vi "SP Find Limit by Parameter.vi"(10 "Parameter":T1={"Stimulus Port"=1, "Response Port"=1} caption="Parameter String" {"Stimulus Port" min=1 step=1; "Response Port" min=1 step=1}, 11 "Limits":T2[](array[typedef]) {"Parameter"."Stimulus Port" min=1 step=1; "Parameter"."Response Port" min=1 step=1}) -> (0 "Found?":bool, 3 "Limits":T2[](array[typedef]) {"Parameter"."Stimulus Port" min=1 step=1; "Parameter"."Response Port" min=1 step=1})   [LabVIEW 2011]
uses:
  TypeDefs/SP Limit.ctl
  TypeDefs/SP Parameter.ctl
  TypeDefs/SP Format.ctl
  TypeDefs/SP Limit Type.ctl
  TypeDefs/SP Limit Point.ctl
  Test Referential Limit.ctl
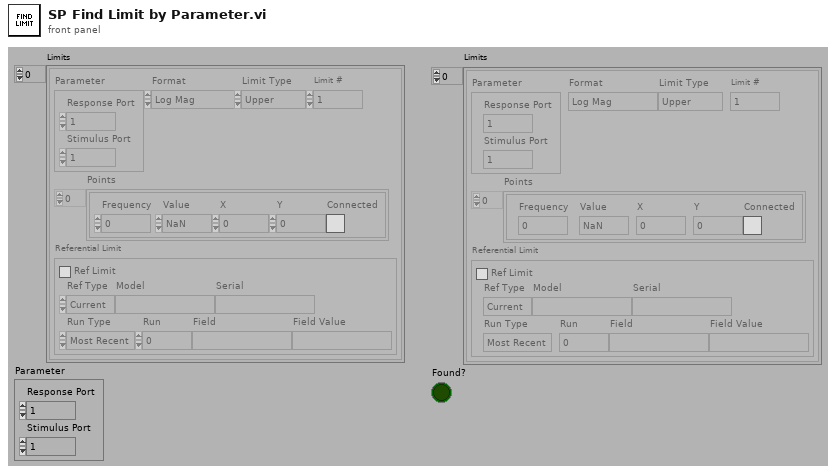
[diagram p1: front panel]
types:
  T1 = typedef "SP Parameter.ctl" = cluster{"Stimulus Port":i8, "Response Port":i8}
  T2 = typedef "SP Limit.ctl" = cluster{"Parameter":T1, "Format":T3, "Limit Type":T4, "Points":T5[], "Referential Limit":T6, "Limit #":i8}
  T3 = typedef "SP Format.ctl" = enum16{"Log Mag", "Lin Mag", "SWR", "Phase", "Expanded Phase", "Delay", "Insertion Loss", "Isolation", "Return Loss"}
  T4 = typedef "SP Limit Type.ctl" = enum16{"Upper", "Lower", "Delta", "Filter", "Referential"}
  T5 = typedef "SP Limit Point.ctl" = cluster{"Frequency":dbl, "Value":dbl, "X":dbl, "Y":dbl, "Connected":bool}
  T6 = typedef "Test Referential Limit.ctl" = cluster{"Ref Limit":bool, "Ref Type":enum16{"Current", "Specify"}, "Model":string, "Serial":string, "Run Type":enum16{"Most Recent", "Run #", "Match Field"}, "Run":i32, "Field":string, "Field Value":string}
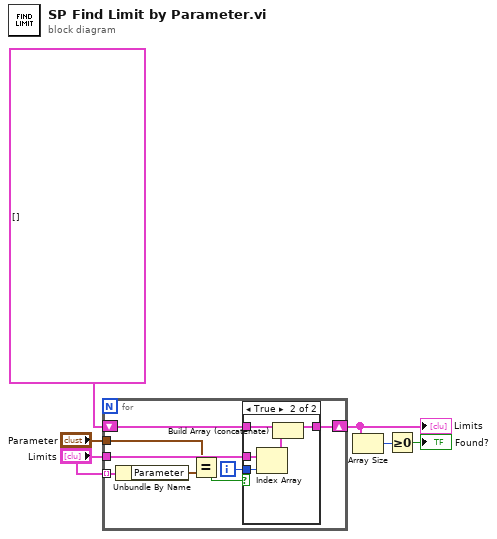
[diagram p0: block diagram]
diagram:
  n1 = for {
    tunnel: "Limits" -> [w14] mode=indexing
    tunnel: "Limits" -> [w13]
    shift-right: [w10] -> w4
    shift-left: T2[] [] ("Limits") -> [w11]
    tunnel: "Parameter" -> [w8]
    i -> [w12]
    n2 = Unbundle By Name(w14) -> ("Parameter"=w9:T1)
    n3 = Equal?(x=w8, y=w9) -> (x = y?=w7:bool)
    n4 = case shown="True" w7 {
      tunnel: w13 -> [_ w20]
      tunnel: w12 -> [_ w19]
      tunnel: w11 -> [w15 w17]
      tunnel: [w15 w16] -> w10
      frame False {
      }
      frame True {
        n5 = Index Array(array=w20, index=w19) -> (element=w18:T2)
        n6 = Build Array (concatenate)(w17, w18) -> (w16:T2[])
      }
    }
  }
  "Limits" <- w4
  n7 = Array Size(array=w4) -> (size(s)=w3:i32)
  n8 = Greater Or Equal To 0?(x=w3) -> (x >= 0?=→"Found?":bool)
